vi "GenerateXML.vi"(6 "static class name":string, 7 "Class version":T1, 8 "Class data as XML":string, 9 "Private data as XML":string, 10 "Parent XML After Child":string, 11 "Parent XML Before Child":string) -> (0 "After Child":string, 1 "Object as XML":string, 3 "Before Child":string)   [LabVIEW 2020, in "OpenG_Object.lvclass"]
doc: "Constructs flattened object XML output by combining XML inputs."
uses:
  OpenG_Object.lvclass
panel:
  # "Please visit http://www.OpenG.org to learn about the\nOpen Source LabVIEW software movement.\n\nNOTICE -- YOU MUST LEAVE THIS NOTICE IN PLACE.  PER THE TERMS OF THE LICENSE BELOW, YOU MAY SUBLICENSE THIS SOFTWARE \nIN ANY WAY THAT DOES NOT CONFLICT WITH THIS LICENSE.\n\n### BSD License (http://www.opensource.org/licenses/bsd-license.php) Begin ###\n\nCopyright (c) 2007, Tomi Maila\nCopyright (c) 2007, Endevo AB\n\n\nAll rights reserved.\n\nRedistribution and use in source and binary forms, with or without modification, are permitted provided that the following conditions are met:\n\n    * Redistributions of source code must retain the above copyright notice, this list of conditions and the following disclaimer.\n    * Redistributions in binary form must reproduce the above copyright notice, this list of conditions and the following disclaimer in the \n       documentation and/or other materials provided with the distribution.\n    * Neither the name of Endevo AB nor the names of the contributors may be used to endorse or promote products derived\n       from this software without specific prior written permission.\n\nTHIS SOFTWARE IS PROVIDED BY THE COPYRIGHT HOLDERS AND CONTRIBUTORS \"AS IS\" AND ANY EXPRESS OR IMPLIED WARRANTIES, \nINCLUDING, BUT NOT LIMITED TO, THE IMPLIED WARRANTIES OF MERCHANTABILITY AND FITNESS FOR A PARTICULAR PURPOSE ARE \nDISCLAIMED. IN NO EVENT SHALL THE COPYRIGHT OWNER OR CONTRIBUTORS BE LIABLE FOR ANY DIRECT, INDIRECT, INCIDENTAL,\n SPECIAL, EXEMPLARY, OR CONSEQUENTIAL DAMAGES (INCLUDING, BUT NOT LIMITED TO, PROCUREMENT OF SUBSTITUTE GOODS OR \nSERVICES; LOSS OF USE, DATA, OR PROFITS; OR BUSINESS INTERRUPTION) HOWEVER CAUSED AND ON ANY THEORY OF LIABILITY, \nWHETHER IN CONTRACT, STRICT LIABILITY, OR TORT (INCLUDING NEGLIGENCE OR OTHERWISE) ARISING IN ANY WAY OUT OF THE USE \nOF THIS SOFTWARE, EVEN IF ADVISED OF THE POSSIBILITY OF SUCH DAMAGE.\n\n### BSD License End ###"
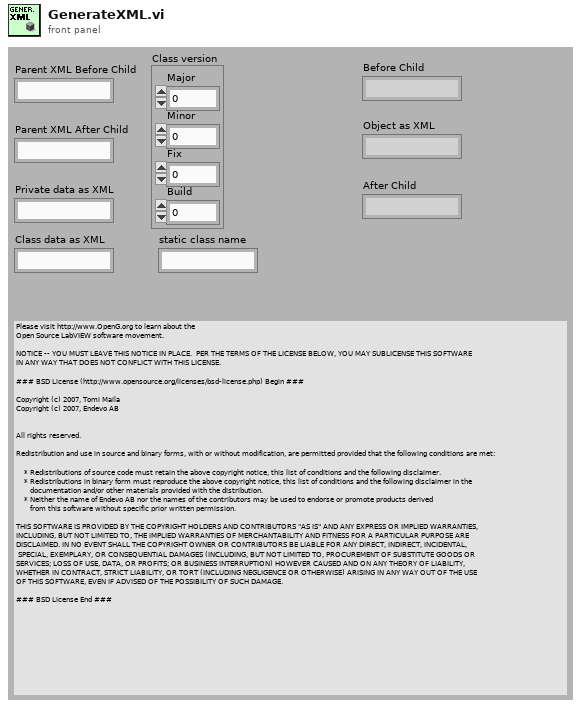
[diagram p1: front panel]
types:
  T1 = cluster{"Major":u16, "Minor":u16, "Fix":u16, "Build":u16}
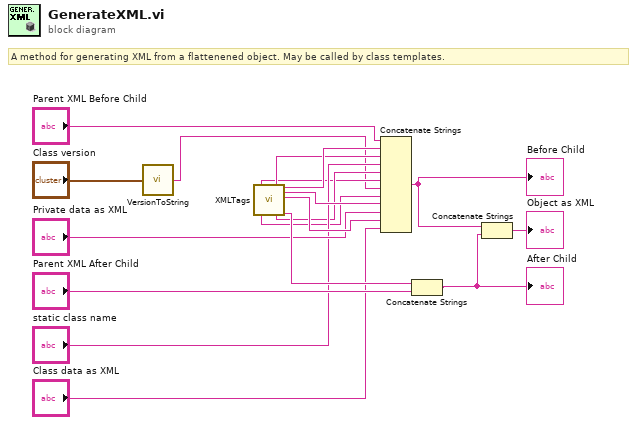
[diagram p0: block diagram]
diagram:
  # "A method for generating XML from a flattenened object. May be called by class templates."
  n1 = call "VersionToString.vi"("Version"="Class version") -> ("Version as string"=w3:string)
  n2 = call "XMLTags.vi"() -> ("<Version>"=w4:string, "</Version>"=w2:string, "<Type>"=w7:string, "</Type>"=w5:string, "<Class>"=w9:string, "<PrivateData>"=w11:string, "</PrivateData>"=w13:string, "</Class>"=w16:string)  [unwired: 4 in, 8 out]
  n3 = Concatenate Strings("Parent XML Before Child", w9, w7, "static class name", w5, w4, w3, w2, w11, "Private data as XML", w13, "Class data as XML") -> (w15:string)
  "Before Child" <- w15
  n4 = Concatenate Strings(w16, "Parent XML After Child") -> (w17:string)
  "After Child" <- w17
  n5 = Concatenate Strings(w15, w17) -> (→"Object as XML":string)
